vi "DSF.Engine.Memory.Transfer.Set ID.vi"(8 "error in (no error)":errorcluster, 10 "id":i32, 11 "Transfer in":refnum<class "DSF.Engine.Memory.Transfer.lvclass">) -> (0 "error out":errorcluster, 3 "Transfer out":refnum<class "DSF.Engine.Memory.Transfer.lvclass">)   [LabVIEW 2016, in "DSF.Engine.lvlib" / "DSF.Engine.Memory.Transfer.lvclass"]
uses:
  DSF.Engine.Memory.Transfer.lvclass
  DSF.Engine.Memory.Transfer.lvclass/DSF.Engine.Memory.Transfer.ctl
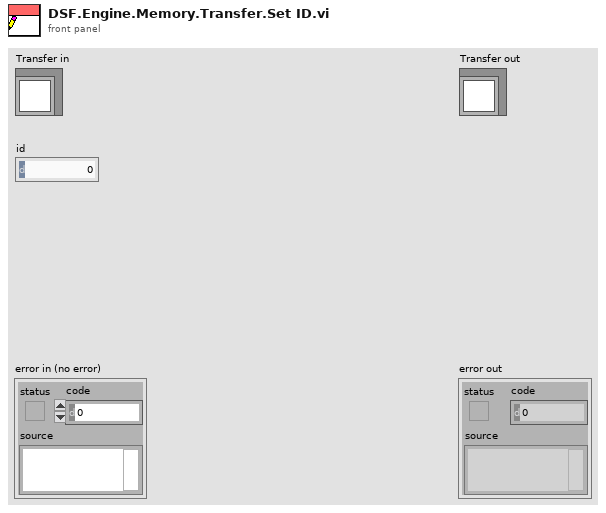
[diagram p1: front panel]
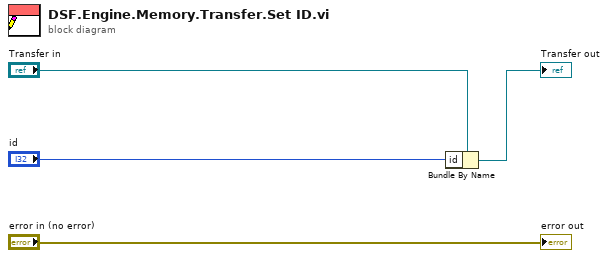
[diagram p0: block diagram]
diagram:
  n1 = Bundle By Name(cluster="Transfer in", "id"="id") -> (→"Transfer out":refnum<class "DSF.Engine.Memory.Transfer.lvclass">)
  "error out" <- "error in (no error)"
